vi "test High Priority Data - RT-RT.vi"(8 "error in (no error)":errorcluster, 11 "BC Async SubRoutines in":refnum<class "BC Async SubRoutines.lvclass">) -> (0 "error out":errorcluster, 3 "BC Async SubRoutines out":refnum<class "BC Async SubRoutines.lvclass">)   [LabVIEW 2016, in "BC Async SubRoutines.lvclass"]
uses:
  BC Async SubRoutines.lvclass
  PPLs/FPGA Interface.lvlibp/FPGA Interface/FPGA Interface.lvclass
  Bus Controller/Bus Controller.lvclass
  1553 Component/1553 Component.lvclass
  Frames & Messages/TypeDefs/Message Control.ctl
  BCI-1553 API.lvlib
  Frames & Messages/TypeDefs/Command Config.ctl
  Frames & Messages/TypeDefs/Async Message Config.ctl
  Frames & Messages/Async RT-RT Message/Async RT-RT Message.lvclass
  Frames & Messages/TypeDefs/Async RT-RT Message Config.ctl
  Frames & Messages/TypeDefs/Command Word Count.ctl
  Frames & Messages/TypeDefs/Command SubAddress.ctl
  Frames & Messages/TypeDefs/Command Terminal Address.ctl
  Frames & Messages/TypeDefs/Command Type.ctl
  Dependencies/FPGA Interface/FPGA Interface.lvclass
  D:/R&D/cRIO 1553 2016/Windows/Frames & Messages/Async Message/Async Message.lvclass
panel:
  out "Data":u16[](array[numeric]) format="%04x"
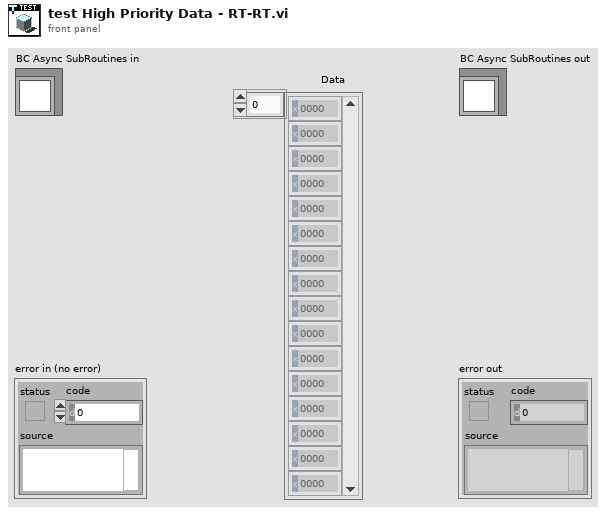
[diagram p1: front panel]
types:
  T1 = typedef "BCI-1553 API.lvlib/Async RT-RT Message Config.ctl" = cluster{"Tx Command Config":T2}
  T2 = typedef "BCI-1553 API.lvlib/Command Config.ctl" = cluster{"Command Type":enum16{"Transmit", "Receive"}, "Terminal Address (0-30)":u16, "SubAddress (1-30)":u16, "WC/MC (1-32)":u16, "Command Data":u16[]}
  T3 = typedef "BCI-1553 API.lvlib/Command Config.ctl" = cluster{"Command Type":T4, "Terminal Address":T5, "SubAddress":T6, "Word Count\\Mode Code":T7, "Command Data":u16[]}
  T4 = typedef "BCI-1553 API.lvlib/Command Type.ctl" = enum16{"Transmit", "Receive"}
  T5 = typedef "BCI-1553 API.lvlib/Command Terminal Address.ctl" = enum16{"0", "1", "2", "3", "4", "5", "6", "7", "8", "9", "10", "11", "12", "13", "14", "15", "16", "17", "18", "19", "20", "21", "22", "23", "24", "25", "26", "27", "28", "29", "30", "Broadcast"}
  T6 = typedef "BCI-1553 API.lvlib/Command SubAddress.ctl" = enum16{"Mode Code", "1", "2", "3", "4", "5", "6", "7", "8", "9", "10", "11", "12", "13", "14", "15", "16", "17", "18", "19", "20", "21", "22", "23", "24", "25", "26", "27", "28", "29", "30"}
  T7 = typedef "BCI-1553 API.lvlib/Command Word Count.ctl" = enum16{"1", "2", "3", "4", "5", "6", "7", "8", "9", "10", "11", "12", "13", "14", "15", "16", "17", "18", "19", "20", "21", "22", "23", "24", "25", "26", "27", "28", "29", "30", "31", "32"}
  T8 = typedef "BCI-1553 API.lvlib/Async Message Config.ctl" = cluster{"Group":i32, "High Priority":bool, "Time to Next Msg (100 us)":u16, "Command Config":T3, "Message Control":T9}
  T9 = typedef "BCI-1553 API.lvlib/Message Control.ctl" = cluster{"MC17 Time Sync":bool, "Error Mask":bool, "Service Request Mask":bool, "Busy Mask":bool, "SubSystem Flag Mask":bool, "Terminal Flag Mask":bool, "Reserved Mask":bool, "Retry":bool, "Bus A / !Bus B":bool, "Self-Test Loopback":bool, "Broadcast Mask":bool, "EoM Interrupt":bool, "Mode Code Format":bool, "Broadcast Format":bool, "RT-RT Format":bool}
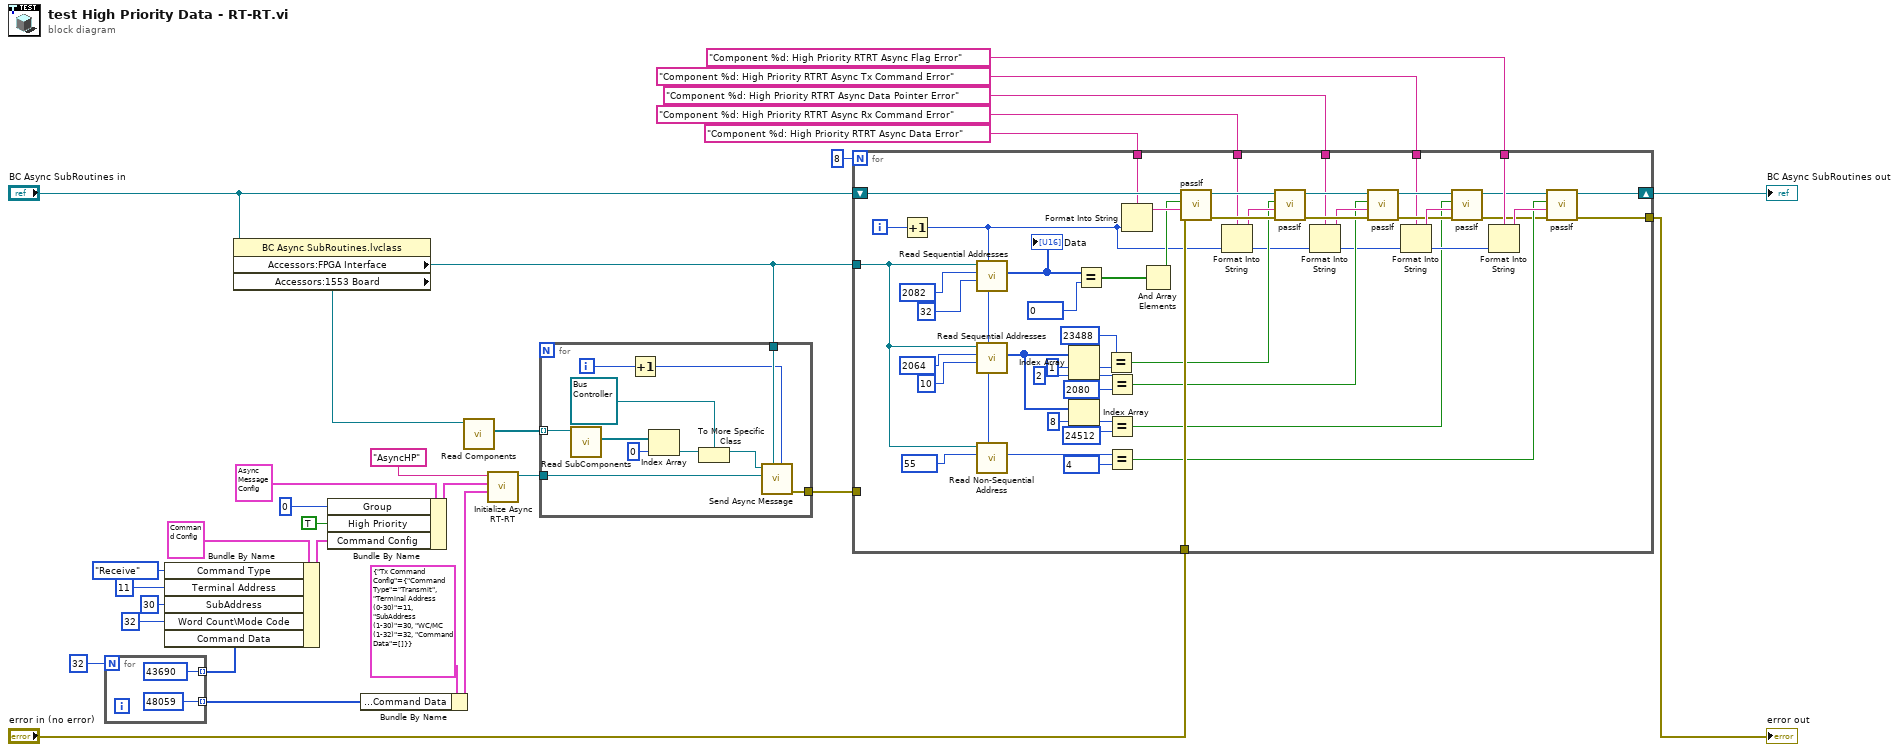
[diagram p0: block diagram]
diagram:
  n1 = for {
    N: 32 -> [_]
    tunnel: [u16 43690] -> w17 mode=indexing
    tunnel: [u16 48059] -> w2 mode=indexing
  }
  n2 = Bundle By Name(cluster=T3 {"Command Type"=enum."Transmit", "Terminal Address"=enum."0", "SubAddress"=enum."Mode Code", "Word Count\\Mode Code"=enum."1", "Command Data"=[]} ("Command Config"), "Command Type"=enum16{"Transmit", "Receive"}."Receive", "Terminal Address"=u16 11 ("Terminal Address (0-30)"), "SubAddress"=u16 30 ("SubAddress (1-30)"), "Word Count\\Mode Code"=u16 32 ("WC/MC (1-32)"), "Command Data"=w17) -> (w24:T3)
  n3 = property class="BC Async SubRoutines.lvclass"(reference="BC Async SubRoutines in") -> ("Accessors:FPGA Interface"=w16:refnum<class "FPGA Interface.lvclass">, "Accessors:1553 Board"=w29:refnum<class "1553 Board.lvclass">)  [unwired: 1 in, 2 out]
  n4 = Bundle By Name(cluster=T8 {"Group"=0, "High Priority"=FALSE, "Time to Next Msg (100 us)"=0, "Command Config"={"Command Type"=enum."Transmit", "Terminal Address"=enum."0", "SubAddress"=enum."Mode Code", "Word Count\\Mode Code"=enum."1", "Command Data"=[]}, "Message Control"={"MC17 Time Sync"=FALSE, "Error Mask"=FALSE, "Service Request Mask"=FALSE, "Busy Mask"=FALSE, "SubSystem Flag Mask"=FALSE, "Terminal Flag Mask"=FALSE, "Reserved Mask"=FALSE, "Retry"=FALSE, "Bus A / !Bus B"=FALSE, "Self-Test Loopback"=FALSE, "Broadcast Mask"=FALSE, "EoM Interrupt"=FALSE, "Mode Code Format"=FALSE, "Broadcast Format"=FALSE, "RT-RT Format"=FALSE}} ("Async Message Config"), "Group"=0, "High Priority"=TRUE, "Command Config"=w24) -> (w5:T8)
  n5 = Bundle By Name(cluster=T1 {"Tx Command Config"={"Command Type"=enum."Transmit", "Terminal Address (0-30)"=11, "SubAddress (1-30)"=30, "WC/MC (1-32)"=32, "Command Data"=[]}} ("RT-RT Async Message Config"), "Tx Command Config.Command Data"=w2) -> (w3:T1)
  n6 = call "Read Components.vi"("1553 Board in"=w29) -> ("Components"=w28:refnum<class "1553 Component.lvclass">[])  [unwired: 8 in, 2 out]
  n7 = call "Initialize Async RT-RT.vi"("Transmit Message Config"=w3, "Receive Message Config"=w5, "ID"="AsyncHP") -> ("Async RT-RT Message out"=w6:refnum<class "Async RT-RT Message.lvclass">)  [unwired: 7 in, 1 out]
  n8 = for {
    tunnel: w28 -> [w44] mode=indexing
    tunnel: w6 -> [w38]
    tunnel: w16 -> [w37]
    tunnel: [w34] -> w15
    i -> [w36]
    n9 = call "Read SubComponents.vi"("1553 Component in"=w44) -> ("SubComponents"=w43:refnum<class "1553 SubComponent.lvclass">[])  [unwired: 8 in, 2 out]
    n10 = Increment(x=w36) -> (x+1=w35:i32)
    n11 = Index Array(array=w43, index=0) -> (element=w41:refnum<class "1553 SubComponent.lvclass">)
    n12 = To More Specific Class(target class=refnum<class "Bus Controller.lvclass"> refnum ("SLSC 1553 API.lvlib:Bus Controller.lvclass"), reference=w41) -> (specific class reference=w39:refnum<class "Bus Controller.lvclass">)  [unwired: 1 in, 1 out]
    n13 = call-dynamic "Send Async Message.vi"("Component ID"=w35, "FPGA Interface"=w37, "Async Message"=w38, "Bus Controller in"=w39) -> ("error out"=w34:errorcluster)  [unwired: 6 in, 1 out]
  }
  n14 = for {
    N: 8 -> [_]
    tunnel: w16 -> [w76]
    shift-right: [w72] -> w10
    shift-left: "BC Async SubRoutines in" -> [w93]
    tunnel: "error in (no error)" -> [w92]
    tunnel: [w69] -> w9
    tunnel: "Component %d: High Priority RTRT Async Data Error" ("custom report message (\"\")") -> [w91]
    tunnel: w15 -> [_]
    tunnel: "Component %d: High Priority RTRT Async Rx Command Error" ("custom report message (\"\")") -> [w68]
    tunnel: "Component %d: High Priority RTRT Async Data Pointer Error" ("custom report message (\"\")") -> [w67]
    tunnel: "Component %d: High Priority RTRT Async Flag Error" ("custom report message (\"\")") -> [w66]
    tunnel: "Component %d: High Priority RTRT Async Tx Command Error" ("custom report message (\"\")") -> [w46]
    i -> [w94]
    n15 = Increment(x=w94) -> (x+1=w47:i32)
    n16 = call-dynamic "Read Sequential Addresses.vi"("Target IC (1-8)"=w47, "Addresses to Read"=u16 32, "Starting Address"=u16 2082, "FPGA Interface in"=w76) -> ("Data"=w84:u16[])  [unwired: 6 in, 1 out]
    "Data" <- w84
    n17 = call-dynamic "Read Sequential Addresses.vi"("Target IC (1-8)"=w47, "Addresses to Read"=u16 10, "Starting Address"=u16 2064, "FPGA Interface in"=w76) -> ("Data"=w56:u16[])  [unwired: 6 in, 1 out]
    n18 = call-dynamic "Read Non-Sequential Address.vi"("Target IC (1-8)"=w47, "Address"=u16 55, "FPGA Interface in"=w76) -> ("Data"=w57:u16)  [unwired: 7 in, 1 out]
    n19 = Index Array(array=w56, index #1=1 ("index"), index #2=2 ("index")) -> (element #1=w78:u16, element #2=w58:u16)
    n20 = Index Array(array=w56, index=8) -> (element=w54:u16)
    n21 = Equal?(x=w84, y=u16 0) -> (x = y?=w82:bool[])
    n22 = Equal?(x=u16 23488, y=w78) -> (x = y?=w62:bool)
    n23 = Equal?(x=w58, y=u16 2080) -> (x = y?=w61:bool)
    n24 = Equal?(x=w54, y=u16 24512) -> (x = y?=w45:bool)
    n25 = Equal?(x=w57, y=u16 4) -> (x = y?=w60:bool)
    n26 = Format Into String(format string=w91, w47) -> (resulting string=w90:string)  [unwired: 2 in, 1 out]
    n27 = And Array Elements(Boolean array=w82) -> (logical AND=w88:bool)
    n28 = call-dynamic "passIf.vi"("error in (no error)"=w92, "message (\"\")"=w90, "pass"=w88, "TestCase in"=w93) -> ("error out"=w71:errorcluster, "TestCase out"=w73:refnum<class "BC Async SubRoutines.lvclass">)  [unwired: 6 in]
    n29 = Format Into String(format string=w68, w47) -> (resulting string=w63:string)  [unwired: 2 in, 1 out]
    n30 = call-dynamic "passIf.vi"("error in (no error)"=w71, "message (\"\")"=w63, "pass"=w62, "TestCase in"=w73) -> ("error out"=w70:errorcluster, "TestCase out"=w74:refnum<class "BC Async SubRoutines.lvclass">)  [unwired: 6 in]
    n31 = Format Into String(format string=w67, w47) -> (resulting string=w64:string)  [unwired: 2 in, 1 out]
    n32 = call-dynamic "passIf.vi"("error in (no error)"=w70, "message (\"\")"=w64, "pass"=w61, "TestCase in"=w74) -> ("error out"=w49:errorcluster, "TestCase out"=w51:refnum<class "BC Async SubRoutines.lvclass">)  [unwired: 6 in]
    n33 = Format Into String(format string=w46, w47) -> (resulting string=w52:string)  [unwired: 2 in, 1 out]
    n34 = call-dynamic "passIf.vi"("error in (no error)"=w49, "message (\"\")"=w52, "pass"=w45, "TestCase in"=w51) -> ("error out"=w48:errorcluster, "TestCase out"=w50:refnum<class "BC Async SubRoutines.lvclass">)  [unwired: 6 in]
    n35 = Format Into String(format string=w66, w47) -> (resulting string=w65:string)  [unwired: 2 in, 1 out]
    n36 = call-dynamic "passIf.vi"("error in (no error)"=w48, "message (\"\")"=w65, "pass"=w60, "TestCase in"=w50) -> ("error out"=w69:errorcluster, "TestCase out"=w72:refnum<class "BC Async SubRoutines.lvclass">)  [unwired: 6 in]
  }
  "error out" <- w9
  "BC Async SubRoutines out" <- w10
